vi "CalibrateUsing2Points.vi"() -> ()   [LabVIEW 2021]
uses:
  <vilib>/userDefined/High Color/IMAQdx.ctl
  include/GlobalVariables.vi
  Other Models/2010/Motion/AbortSingle.vi
  <vilib>/vision/driver/NI_Vision_Acquisition_Software.lvlib
panel:
  out "X2Y2":string
  out "X1Y1":string
  in  "ObjectDetType":T1(ring)
  in  "Gcode2":string="G90\nG1 Z0 F100\nG1 X926.509 Y1005.63 F100//SiR\nG1 Z73.805//SiR\nG1X1301.398 Y999.339 F100//SiOnBPL\nG1Z67.034//SiOnBPL"
  in  "Gcode1":string="G90\nG1 Z0 F100\nG1 X763.262 Y1007.77 F100//SiL\nG1 Z73.805//SiL\nG1X138.057 Y999.293 F100//SiOnBPL\nG1Z67.034//SiOnBPL"
  in  "Operation2":enum16{"JoyStick", "FixedXY"}(ring)
  in  "Operation1":enum16{"JoyStick", "FixedXY"}(ring)
  out "CamX1Y1X2Y2Dist":string
  out "DistanceCam":dbl
  out "CamY 2":dbl
  out "CamX 2":dbl
  out "CamY":dbl
  out "CamX":dbl
  out "error out":errorcluster
  out "XYZU":string
  out "Y2":dbl format="%#_7g"
  out "X2":dbl
  out "Radius 2":dbl
  out "CenterPosition 2":cluster{"X":sgl, "Y":sgl}
  in  "StopJoyStick 2":bool
  out "Image 2":T2(plugin-control)
  out "Y1":dbl format="%#_7g"
  out "X1":dbl
  out "Radius":dbl
  out "CenterPosition":cluster{"X":sgl, "Y":sgl}
  in  "StopJoyStick":bool
  in  "Autofocus":T3={"Enable"=TRUE, "InitialStepSize"=0.05, "Tolerance"=0.02, "Abort"=FALSE} {"Tolerance" format="%#_13g"}
  out "Image":T2(plugin-control)
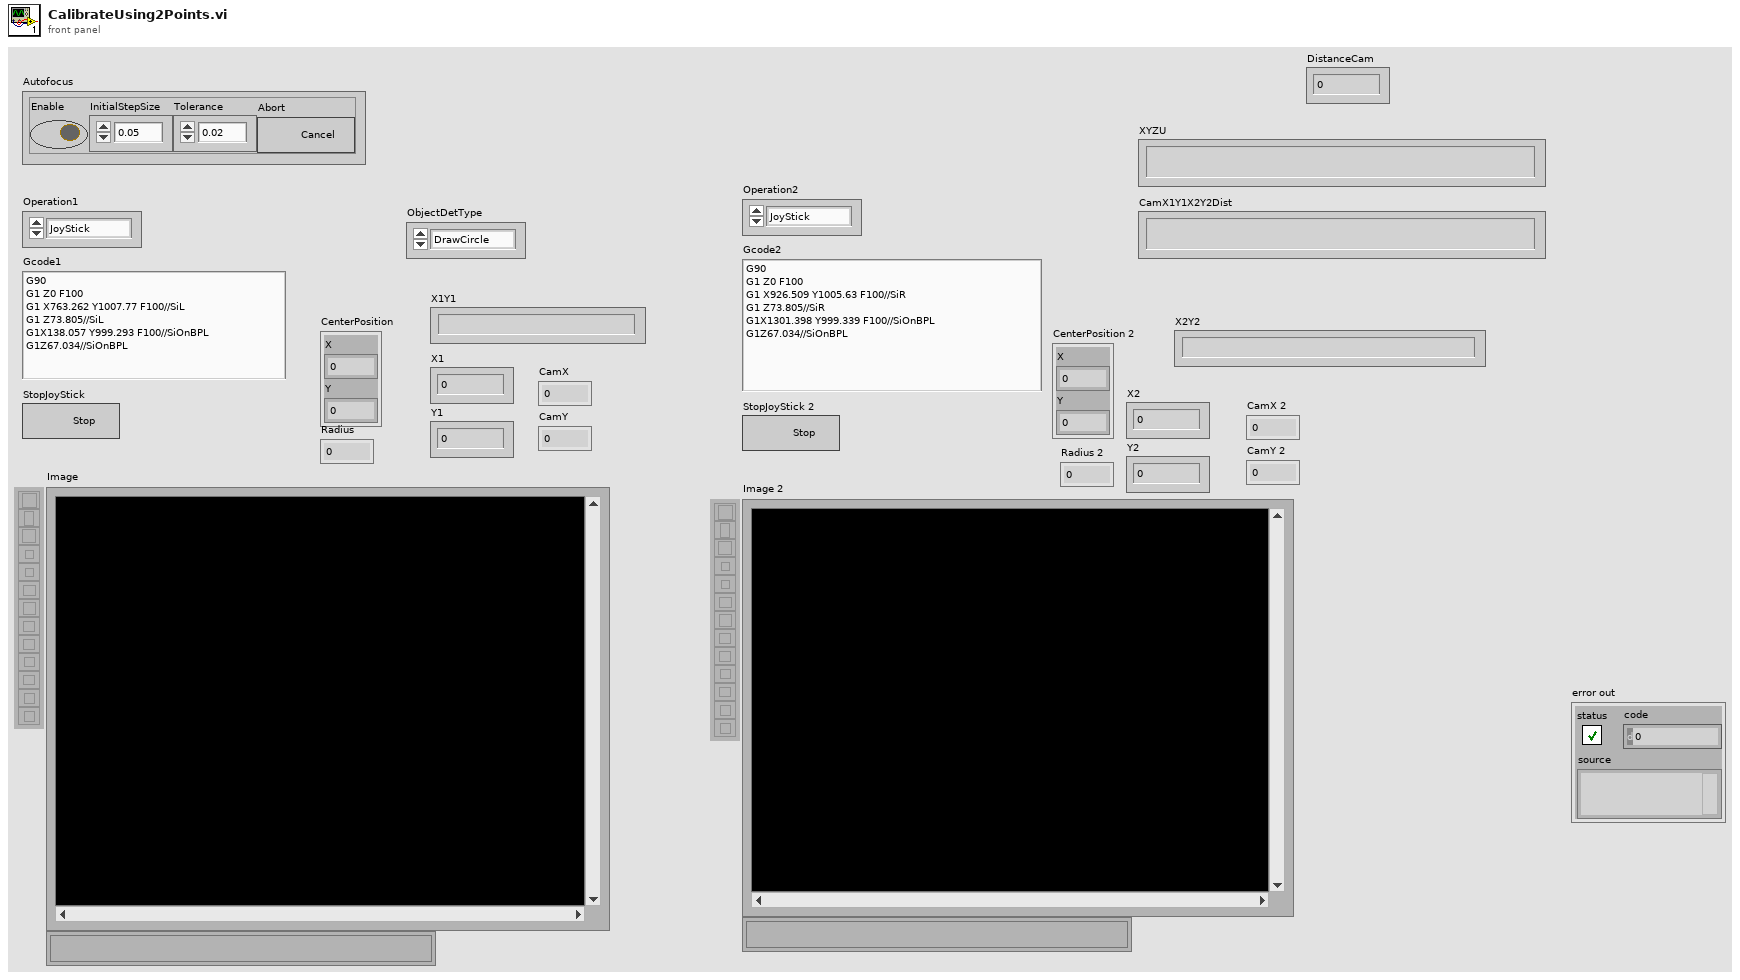
[diagram p1: front panel]
types:
  T1 = enum16{"DrawCircle", "Pattern", "ManualPick", "FidCircle"}
  T2 = typedef "IMAQ Image.ctl" = refnum<image>
  T3 = cluster{"Enable":bool, "InitialStepSize":dbl, "Tolerance":dbl, "Abort":bool}
  T4 = typedef "IMAQdx.ctl" = refnum<k21>
  T5 = typedef "Image Type" = u32
  T6 = typedef "IMAQ Point" = cluster{"X":sgl, "Y":sgl}
  T7 = typedef "IMAQ Circle" = cluster{"Center X":i32, "Center Y":i32, "Inner Radius":i32, "Outer Radius":i32, "Start Angle":dbl, "End Angle":dbl}
  T8 = cluster{"Position":cluster{"X":sgl, "Y":sgl}, "Radius":dbl, "Score":dbl}
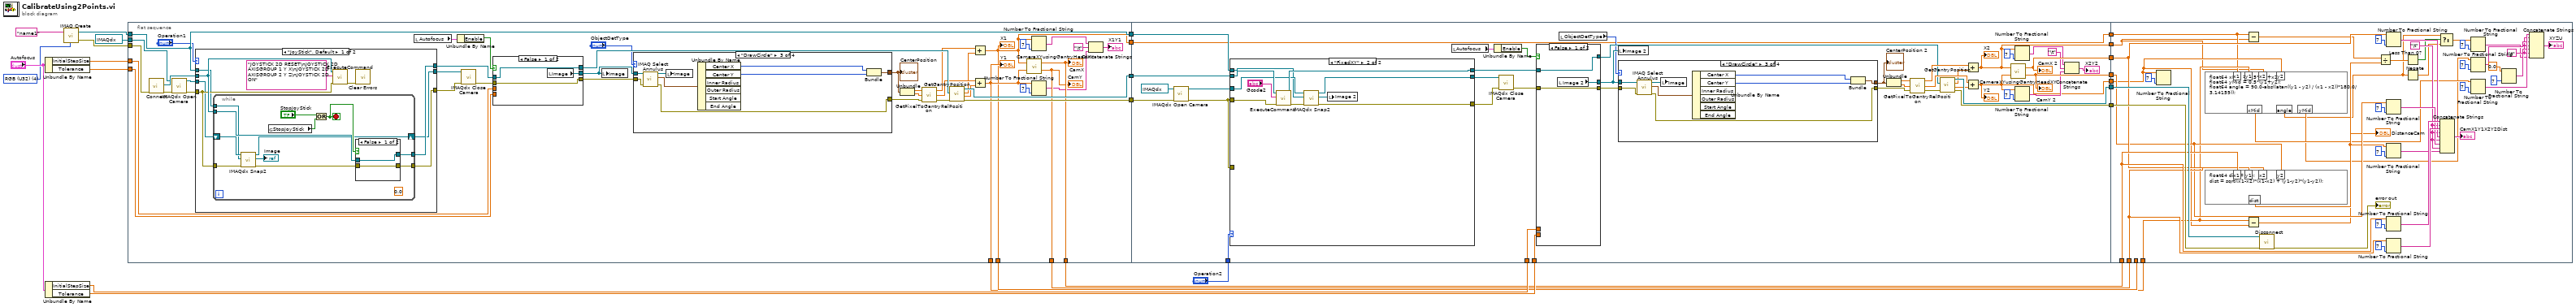
[diagram p0: block diagram]
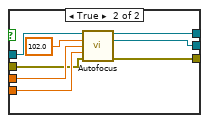
[diagram p2: hidden frame]
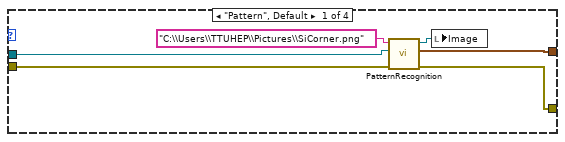
[diagram p3: hidden frame]
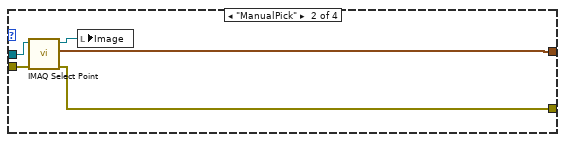
[diagram p4: hidden frame]
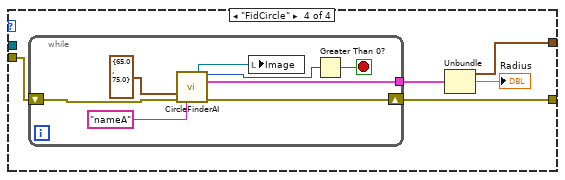
[diagram p5: hidden frame]
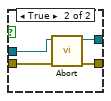
[diagram p6: hidden frame]
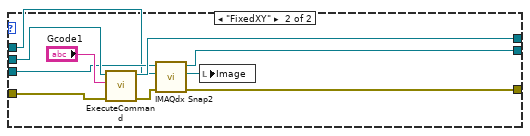
[diagram p7: hidden frame]
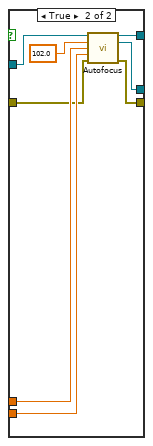
[diagram p8: hidden frame]
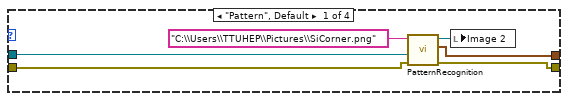
[diagram p9: hidden frame]
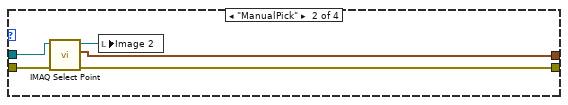
[diagram p10: hidden frame]
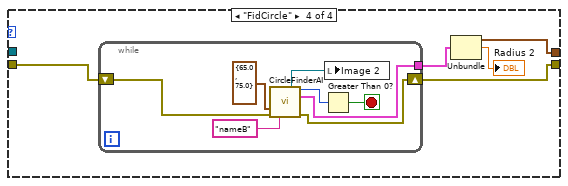
[diagram p11: hidden frame]
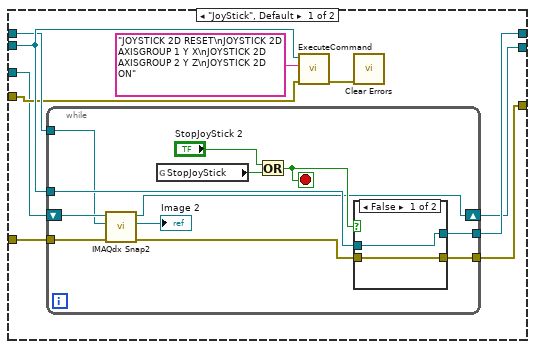
[diagram p12: hidden frame]
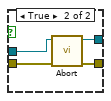
[diagram p13: hidden frame]
diagram:
  w14 = T5 4 items=["Grayscale (U8)", "Grayscale (I16)", "Grayscale (SGL)", "Complex (CSG)", "RGB (U32)", "HSL (U32)", "RGB (U64)", "Grayscale (U16)"] ("Image Type")
  n1 = Unbundle By Name("Autofocus") -> ("InitialStepSize"=w25:dbl, "Tolerance"=w26:dbl)
  n2 = Unbundle By Name("Autofocus") -> ("InitialStepSize"=w21:dbl, "Tolerance"=w20:dbl)
  n3 = call "IMAQ Create"("Image Name"="name1" ("ImageName"), "Image Type"=w14) -> ("New Image"=w13:T2, "error out"=w11:errorcluster)  [unwired: 3 in]
  n4 = flat-sequence {
    tunnel: w26 -> [w67]
    tunnel: w25 -> [w66]
    tunnel: [w63] -> w23
    tunnel: [w62] -> w22
    tunnel: [w27] -> w17
    tunnel: [w53] -> w16
    tunnel: w13 -> [w61]
    tunnel: [w61] -> w12
    tunnel: w11 -> [w56]
    tunnel: T4 "cam1" ("Camera") -> [w57]
    tunnel: [w60] -> w5
    tunnel: [w59] -> w4
    tunnel: [w27] -> w1
    tunnel: w23 -> [w188]
    tunnel: w22 -> [w184]
    tunnel: w21 -> [w187]
    tunnel: w20 -> [w186]
    tunnel: [w172] -> w19
    tunnel: [w171] -> w18
    tunnel: w12 -> [w185]
    tunnel: [w183] -> w9
    tunnel: [w182] -> w8
    tunnel: [w181] -> w7
    tunnel: [w180] -> w6
    tunnel: "Operation2" -> [w179]
    tunnel: [w148] -> w2
    tunnel: w1 -> [w148]
    tunnel: w19 -> [w277]
    tunnel: w18 -> [w279]
    tunnel: w17 -> [_]
    tunnel: w16 -> [w280]
    tunnel: w9 -> [w314]
    tunnel: w8 -> [w313]
    tunnel: w7 -> [w291]
    tunnel: w6 -> [w290]
    tunnel: w5 -> [w293]
    tunnel: w4 -> [w292]
    tunnel: w2 -> [w278]
    frame #0 {
      n5 = call "Connect.vi"("error in (no error)"=w56) -> ("error out"=w64:errorcluster, "controller"=w65:refnum<k24>)  [unwired: 9 in]
      n6 = call <vilib>:"IMAQdx Open Camera.vi"("error in"=w64, "Session In"=w57) -> ("error out"=w32:errorcluster, "Session Out"=w33:T4)  [unwired: 8 in]
      n7 = case shown="\"JoyStick\", Default" "Operation1" {
        tunnel: w65 -> [w118 w147]
        tunnel: [w116 w145] -> w48
        tunnel: w32 -> [w115 w146]
        tunnel: w61 -> [w114 w139]
        tunnel: w33 -> [w113 w143]
        tunnel: [w112 w141] -> w36
        tunnel: [w111 w140] -> w35
        frame "JoyStick", Default {
          n8 = while {
            tunnel: w118 -> [w131]
            tunnel: [w130] -> w112
            tunnel: [w129] -> w116
            tunnel: w115 -> [w125]
            shift-right: [w123] -> w111
            shift-left: w113 -> [w122]
            tunnel: w114 -> [w120]
            stop <- w126 stop-if-true
            (unwired) sgl 0.0 ("Rotate (degrees)")
            n9 = call <vilib>:"IMAQdx Snap2.vi"("error in"=w125, "Image In"=w120, "Session In"=w122) -> ("error out"=w121:errorcluster, "Image Out"=→"Image":T2, "Session Out"=w123:T4)  [unwired: 6 in]
            n10 = global read "GlobalVariables.vi" "StopJoyStick"() -> (w127:bool)
            n11 = Or(x="StopJoyStick", y=w127) -> (x .or. y?=w126:bool)
            n12 = case shown="False" w126 {
              tunnel: w131 -> [w133 w137]
              tunnel: w121 -> [w132 w136]
              tunnel: [w132 w135] -> w130
              tunnel: [w133 w134] -> w129
              frame False {
              }
              frame True {
                n13 = call-poly "Abort.vi"("error in (no error)"=w136, "controller in"=w137) -> ("error out"=w135:errorcluster, "controller out"=w134:refnum<k24>)  [unwired: 8 in]
              }
            }
          }
          n14 = call "ExecuteCommand.vi"("error in (no error)"=w115, "Command Code"="JOYSTICK 2D RESET\nJOYSTICK 2D AXISGROUP 1 Y X\nJOYSTICK 2D AXISGROUP 2 Y Z\nJOYSTICK 2D ON", "controller in"=w118) -> ("error out"=w117:errorcluster)  [unwired: 6 in, 2 out]
          n15 = call <vilib>:"Clear Errors.vi"("error in (no error)"=w117) -> ()  [unwired: 5 in, 2 out]
        }
        frame "FixedXY" {
          n16 = call "ExecuteCommand.vi"("error in (no error)"=w146, "Command Code"="Gcode1", "controller in"=w147) -> ("error out"=w142:errorcluster, "controller out"=w145:refnum<k24>)  [unwired: 6 in, 1 out]
          n17 = call <vilib>:"IMAQdx Snap2.vi"("error in"=w142, "Image In"=w139, "Session In"=w143) -> ("error out"=w141:errorcluster, "Image Out"=w138:T2, "Session Out"=w140:T4)  [unwired: 6 in]
          n18 = local write "Image"(w138) -> ()
        }
      }
      n19 = local read "Autofocus"() -> (w29:T3)
      n20 = Unbundle By Name(w29) -> ("Enable"=w28:bool)
      n21 = call <vilib>:"IMAQdx Close Camera.vi"("error in"=w36, "Session In"=w35) -> ("error out"=w34:errorcluster)  [unwired: 9 in]
      n22 = case shown="False" w28 {
        tunnel: w67 -> [_ w77]
        tunnel: w66 -> [_ w76]
        tunnel: w48 -> [w69 w75]
        tunnel: [w70 w74] -> w47
        tunnel: [w69 w73] -> w46
        tunnel: w34 -> [w70 w72]
        tunnel: [w68 w71] -> w31
        frame False {
          n23 = local read "Image"() -> (w68:T2)
        }
        frame True {
          n24 = call "Autofocus.vi"("controller in"=w75, "SafeMaxZ"=102.0, "InitialStepSize"=w76, "Tolerance"=w77, "error in (no error)"=w72) -> ("controller out"=w73:refnum<k24>, "Image"=w71:T2, "error out"=w74:errorcluster)  [unwired: 5 in, 3 out]
        }
      }
      n25 = local write "Image"(w31) -> ()
      n26 = case shown="\"DrawCircle\"" "ObjectDetType" {
        tunnel: w47 -> [w79 w86 w96 w102]
        tunnel: [w80 w88 w90 w99] -> w45
        tunnel: [w81 w87 w94 w98] -> w42
        tunnel: w31 -> [w83 w89 w97 _]
        frame "Pattern", Default {
          n27 = call "PatternRecognition.vi"("error in (no error)"=w79, "ImageIn"=w83, "TemplateFileName"="C:\\Users\\TTUHEP\\Pictures\\SiCorner.png") -> ("error out"=w81:errorcluster, "Position"=w80:cluster{"x":sgl, "y":sgl}, "ImageFoundPattern"=w82:T2)  [unwired: 3 in, 2 out]
          n28 = local write "Image"(w82) -> ()
        }
        frame "ManualPick" {
          n29 = call "IMAQ Select Point"("error in (no error)"=w86, "Image In"=w89) -> ("error out"=w87:errorcluster, "Point"=w88:T6, "Image Out (duplicate)"=w85:T2)  [unwired: 6 in, 1 out]
          n30 = local write "Image"(w85) -> ()
        }
        frame "DrawCircle" {
          n31 = call "IMAQ Select Annulus"("error in (no error)"=w96, "Image In"=w97) -> ("error out"=w94:errorcluster, "Annulus"=w93:T7, "Image Out (duplicate)"=w95:T2)  [unwired: 6 in, 1 out]
          n32 = local write "Image"(w95) -> ()
          n33 = Unbundle By Name(w93) -> ("Center X"=w92:i32, "Center Y"=w91:i32)  [unwired: 4 out]
          n34 = Bundle("Center X"=w92, "Center Y"=w91) -> (w90:cluster{"Center X":i32, "Center Y":i32})  [unwired: 1 in]
        }
        frame "FidCircle" {
          n35 = while {
            tunnel: [w107] -> w101
            shift-right: [w106] -> w98
            shift-left: w102 -> [w108]
            stop <- w103 stop-if-true
            n36 = call "CircleFinderAI.vi"("Circle Descriptor"=cluster{"Min Radius":dbl, "Max Radius":dbl} {"Min Radius"=65.0, "Max Radius"=75.0}, "error in (no error)"=w108, "Image Name"="nameA") -> ("Image"=w105:T2, "NumCirclesFound"=w104:i32, "Circle0"=w107:T8, "error out"=w106:errorcluster)  [unwired: 7 in, 2 out]
            n37 = local write "Image"(w105) -> ()
            n38 = Greater Than 0?(x=w104) -> (x > 0?=w103:bool)
          }
          n39 = Unbundle(w101) -> ("Position"=w99:cluster{"X":sgl, "Y":sgl}, "Radius"=→"Radius":dbl)  [unwired: 1 out]
        }
      }
      "CenterPosition" <- w45
      n40 = Unbundle(w45) -> ("X"=w44:sgl, "Y"=w43:sgl)
      n41 = call "GetPixelToGantryRelPosition.vi"("error in (no error)"=w42, "PixelY"=w43, "PixelX"=w44) -> ("error out"=w41:errorcluster, "YmmRelGH"=w39:dbl, "XmmRelGH"=w37:dbl)
      n42 = call "GetGantryPosition.vi"("error in (no error)"=w41, "Controller In"=w46) -> ("error out"=w62:errorcluster, "Position Y"=w40:dbl, "Position X"=w38:dbl, "controller out"=w63:refnum<k24>)  [unwired: 3 in, 3 out]
      n43 = Add(x=w37, y=w38) -> (x+y=w27:dbl)
      "X1" <- w27
      n44 = Add(x=w39, y=w40) -> (x+y=w53:dbl)
      "Y1" <- w53
      n45 = call "CameraXYusingGantryHeadXY.vi"("GantryY"=w53, "GantryX"=w27) -> ("CamY"=w59:dbl, "CamX"=w60:dbl)
      "CamX" <- w60
      "CamY" <- w59
      n46 = Number To Fractional String(number=w27, precision (6)=i16 7) -> (F-format string=w52:string)  [unwired: 2 in]
      n47 = Number To Fractional String(number=w53, precision (6)=i16 7) -> (F-format string=w50:string)  [unwired: 2 in]
      n48 = Concatenate Strings(w52, "\t", w50) -> (→"X1Y1":string)
    }
    frame #1 {
      n49 = call <vilib>:"IMAQdx Open Camera.vi"("error in"=w184, "Session In"=T4 "cam1") -> ("error out"=w154:errorcluster, "Session Out"=w153:T4)  [unwired: 8 in]
      n50 = case shown="\"FixedXY\"" w179 {
        tunnel: w188 -> [w241 w268]
        tunnel: [w238 w267] -> w159
        tunnel: [w237 w261] -> w158
        tunnel: [w236 w262] -> w157
        tunnel: w185 -> [w235 w265]
        tunnel: w154 -> [w234 w263]
        tunnel: w154 -> [w233 _]
        tunnel: w153 -> [w232 w266]
        frame "JoyStick", Default {
          n51 = while {
            tunnel: w241 -> [w253]
            tunnel: [w252] -> w236
            tunnel: [w251] -> w238
            shift-right: [w246] -> w237
            shift-left: w232 -> [w247]
            tunnel: w235 -> [w243]
            tunnel: w233 -> [w242]
            stop <- w248 stop-if-true
            n52 = call <vilib>:"IMAQdx Snap2.vi"("error in"=w242, "Image In"=w243, "Session In"=w247) -> ("error out"=w244:errorcluster, "Image Out"=→"Image 2":T2, "Session Out"=w246:T4)  [unwired: 6 in]
            n53 = global read "GlobalVariables.vi" "StopJoyStick"() -> (w249:bool)
            n54 = Or(x="StopJoyStick 2", y=w249) -> (x .or. y?=w248:bool)
            n55 = case shown="False" w248 {
              tunnel: w253 -> [w255 w259]
              tunnel: w244 -> [w254 w258]
              tunnel: [w254 w257] -> w252
              tunnel: [w255 w256] -> w251
              frame False {
              }
              frame True {
                n56 = call-poly "Abort.vi"("error in (no error)"=w258, "controller in"=w259) -> ("error out"=w257:errorcluster, "controller out"=w256:refnum<k24>)  [unwired: 8 in]
              }
            }
          }
          n57 = call "ExecuteCommand.vi"("error in (no error)"=w234, "Command Code"="JOYSTICK 2D RESET\nJOYSTICK 2D AXISGROUP 1 Y X\nJOYSTICK 2D AXISGROUP 2 Y Z\nJOYSTICK 2D ON", "controller in"=w241) -> ("error out"=w240:errorcluster)  [unwired: 6 in, 2 out]
          n58 = call <vilib>:"Clear Errors.vi"("error in (no error)"=w240) -> ()  [unwired: 5 in, 2 out]
        }
        frame "FixedXY" {
          n59 = call "ExecuteCommand.vi"("error in (no error)"=w263, "Command Code"="Gcode2", "controller in"=w268) -> ("error out"=w264:errorcluster, "controller out"=w267:refnum<k24>)  [unwired: 6 in, 1 out]
          n60 = call <vilib>:"IMAQdx Snap2.vi"("error in"=w264, "Image In"=w265, "Session In"=w266) -> ("error out"=w262:errorcluster, "Image Out"=w260:T2, "Session Out"=w261:T4)  [unwired: 6 in]
          n61 = local write "Image 2"(w260) -> ()
        }
      }
      n62 = local read "Autofocus"() -> (w150:T3)
      n63 = Unbundle By Name(w150) -> ("Enable"=w149:bool)
      n64 = call <vilib>:"IMAQdx Close Camera.vi"("error in"=w157, "Session In"=w158) -> ("error out"=w156:errorcluster)  [unwired: 9 in]
      n65 = case shown="False" w149 {
        tunnel: [w190 w199] -> w161
        tunnel: [w191 w198] -> w160
        tunnel: w159 -> [w190 w197]
        tunnel: w187 -> [_ w195]
        tunnel: w186 -> [_ w194]
        tunnel: w156 -> [w191 w193]
        tunnel: [w189 w192] -> w152
        frame False {
          n66 = local read "Image 2"() -> (w189:T2)
        }
        frame True {
          n67 = call "Autofocus.vi"("controller in"=w197, "SafeMaxZ"=102.0, "InitialStepSize"=w195, "Tolerance"=w194, "error in (no error)"=w193) -> ("controller out"=w199:refnum<k24>, "Image"=w192:T2, "error out"=w198:errorcluster)  [unwired: 5 in, 3 out]
        }
      }
      n68 = local read "ObjectDetType"() -> (w151:T1)
      n69 = local write "Image 2"(w152) -> ()
      n70 = case shown="\"DrawCircle\"" w151 {
        tunnel: [w202 w208 w214 w223] -> w165
        tunnel: [w200 w207 w212 w222] -> w162
        tunnel: w160 -> [w203 w209 w215 w219]
        tunnel: w152 -> [w204 w210 w216 _]
        frame "Pattern", Default {
          n71 = call "PatternRecognition.vi"("error in (no error)"=w203, "ImageIn"=w204, "TemplateFileName"="C:\\Users\\TTUHEP\\Pictures\\SiCorner.png") -> ("error out"=w202:errorcluster, "Position"=w200:cluster{"x":sgl, "y":sgl}, "ImageFoundPattern"=w201:T2)  [unwired: 3 in, 2 out]
          n72 = local write "Image 2"(w201) -> ()
        }
        frame "ManualPick" {
          n73 = call "IMAQ Select Point"("error in (no error)"=w209, "Image In"=w210) -> ("error out"=w208:errorcluster, "Point"=w207:T6, "Image Out (duplicate)"=w206:T2)  [unwired: 6 in, 1 out]
          n74 = local write "Image 2"(w206) -> ()
        }
        frame "DrawCircle" {
          n75 = call "IMAQ Select Annulus"("error in (no error)"=w215, "Image In"=w216) -> ("error out"=w214:errorcluster, "Annulus"=w218:T7, "Image Out (duplicate)"=w211:T2)  [unwired: 6 in, 1 out]
          n76 = local write "Image"(w211) -> ()
          n77 = Unbundle By Name(w218) -> ("Center X"=w213:i32, "Center Y"=w217:i32)  [unwired: 4 out]
          n78 = Bundle("Center X"=w213, "Center Y"=w217) -> (w212:cluster{"Center X":i32, "Center Y":i32})  [unwired: 1 in]
        }
        frame "FidCircle" {
          n79 = while {
            tunnel: [w230] -> w220
            shift-right: [w231] -> w223
            shift-left: w219 -> [w229]
            stop <- w224 stop-if-true
            n80 = call "CircleFinderAI.vi"("Circle Descriptor"=cluster{"Min Radius":dbl, "Max Radius":dbl} {"Min Radius"=65.0, "Max Radius"=75.0}, "error in (no error)"=w229, "Image Name"="nameB") -> ("Image"=w227:T2, "NumCirclesFound"=w225:i32, "Circle0"=w230:T8, "error out"=w231:errorcluster)  [unwired: 7 in, 2 out]
            n81 = Greater Than 0?(x=w225) -> (x > 0?=w224:bool)
            n82 = local write "Image 2"(w227) -> ()
          }
          n83 = Unbundle(w220) -> ("Position"=w222:cluster{"X":sgl, "Y":sgl}, "Radius"=→"Radius 2":dbl)  [unwired: 1 out]
        }
      }
      "CenterPosition 2" <- w162
      n84 = Unbundle(w162) -> ("X"=w163:sgl, "Y"=w164:sgl)
      n85 = call "GetPixelToGantryRelPosition.vi"("error in (no error)"=w165, "PixelY"=w164, "PixelX"=w163) -> ("error out"=w166:errorcluster, "YmmRelGH"=w169:dbl, "XmmRelGH"=w167:dbl)
      n86 = call "GetGantryPosition.vi"("error in (no error)"=w166, "Controller In"=w161) -> ("error out"=w182:errorcluster, "Position Y"=w170:dbl, "Position X"=w168:dbl, "controller out"=w183:refnum<k24>)  [unwired: 3 in, 3 out]
      n87 = Add(x=w167, y=w168) -> (x+y=w172:dbl)
      "X2" <- w172
      n88 = Add(x=w169, y=w170) -> (x+y=w171:dbl)
      "Y2" <- w171
      n89 = call "CameraXYusingGantryHeadXY.vi"("GantryY"=w171, "GantryX"=w172) -> ("CamY"=w180:dbl, "CamX"=w181:dbl)
      "CamX 2" <- w181
      "CamY 2" <- w180
      n90 = Number To Fractional String(number=w172, precision (6)=i16 7) -> (F-format string=w176:string)  [unwired: 2 in]
      n91 = Number To Fractional String(number=w171, precision (6)=i16 7) -> (F-format string=w174:string)  [unwired: 2 in]
      n92 = Concatenate Strings(w176, "\t", w174) -> (→"X2Y2":string)
    }
    frame #2 {
      w296 = "\t"
      w282 = "\t"
      n93 = Number To Fractional String(number=w279, precision (6)=i16 7) -> ()  [unwired: 2 in, 1 out]
      n94 = formula code="float64 xMid = 0.5*(x1+x2);\nfloat64 yMid = 0.5*(y1+y2);\nfloat64 angle = 90.0-abs((atan((y1 - y2) / (x1 - x2))*180.0/3.14159));"("x1"=w278, "y1"=w280, "x2"=w277, "y2"=w279) -> ("xMid"=w288:dbl, "yMid"=w287:dbl, "angle"=w271:dbl)
      n95 = formula code="float64 dist = 0.0;\ndist = sqrt((x1-x2)*(x1-x2) + (y1-y2)*(y1-y2));"("x1"=w293, "y1"=w292, "x2"=w291, "y2"=w290) -> ("dist"=w289:dbl)
      "DistanceCam" <- w289
      n96 = Subtract(x=w278, y=w277) -> (x-y=w276:dbl)
      n97 = Subtract(x=w280, y=w279) -> (x-y=w275:dbl)
      n98 = call "Disconnect.vi"("error in (no error)"=w313, "controller"=w314) -> ("error out"=→"error out":errorcluster)  [unwired: 9 in]
      n99 = Divide(x=w276, y=w275) -> (x/y=w274:dbl)
      n100 = Number To Fractional String(number=w291, precision (6)=i16 7) -> (F-format string=w298:string)  [unwired: 2 in]
      n101 = Number To Fractional String(number=w290, precision (6)=i16 7) -> (F-format string=w297:string)  [unwired: 2 in]
      n102 = Number To Fractional String(number=w289, precision (6)=i16 7) -> (F-format string=w295:string)  [unwired: 2 in]
      n103 = Number To Fractional String(number=w293, precision (6)=i16 7) -> (F-format string=w300:string)  [unwired: 2 in]
      n104 = Number To Fractional String(number=w292, precision (6)=i16 7) -> (F-format string=w299:string)  [unwired: 2 in]
      n105 = Less Than 0?(x=w274) -> (x < 0?=w273:bool)
      n106 = Negate(x=w271) -> (-x=w270:dbl)
      n107 = Select(t=w271, s=w273, f=w270) -> (s? t:f=w272:dbl)
      n108 = Concatenate Strings(w300, w296, w299, w296, w298, w296, w297, w296, w295) -> (→"CamX1Y1X2Y2Dist":string)
      n109 = Number To Fractional String(number=w272, precision (6)=i16 7) -> (F-format string=w281:string)  [unwired: 2 in]
      n110 = Number To Fractional String(number=w287, precision (6)=i16 7) -> (F-format string=w285:string)  [unwired: 2 in]
      n111 = Number To Fractional String(number=w288, precision (6)=i16 7) -> (F-format string=w286:string)  [unwired: 2 in]
      n112 = Number To Fractional String(number=0.0, precision (6)=i16 7) -> (F-format string=w283:string)  [unwired: 2 in]
      n113 = Concatenate Strings(w286, w282, w285, w282, w283, w282, w281) -> (→"XYZU":string)
    }
  }
